vi "Get Shared Variable IP Info.vi"(8 "error in (no error)":errorcluster, 11 "IP Address":string) -> (0 "error out":errorcluster, 3 "Sh Var Data Array":T1[](array[typedef]))   [LabVIEW 2012, in "Shared Variable Custom Device.lvlib"]
uses:
  Shared Variable Custom Device.lvlib
  RTMs/Tree Data.ctl
  <vilib>/Utility/VariantDataType/Type.ctl
  Shared/Shared Variable Globals.vi
  <resource>/objmgr/ni.var.rc
  <vilib>/Utility/VariantDataType/VariantType.lvlib
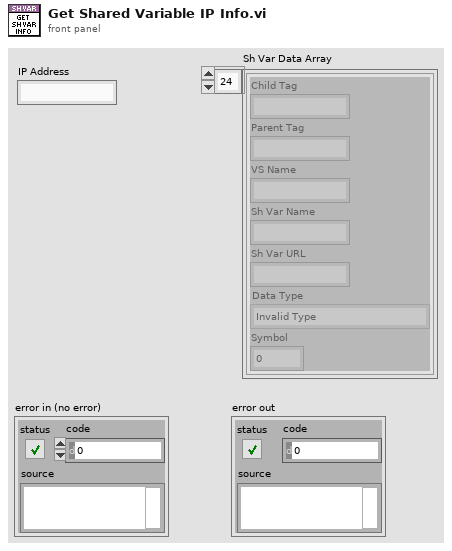
[diagram p1: front panel]
types:
  T1 = typedef "Shared Variable Custom Device.lvlib/Tree Data.ctl" = cluster{"Child Tag":string, "Parent Tag":string, "VS Name":string, "Sh Var Name":string, "Sh Var URL":string, "Data Type":T2, "Symbol":i32}
  T2 = typedef "VariantType.lvlib/Type.ctl" = enum8{"Invalid Type", "Void", "I8", "I16", "I32", "I64", "U8", "U16", "U32", "U64", "Single Float", "Double Float", "Extended Float", "Single Complex", "Double Complex", "Extended Complex", "Enum U8", "Enum U16", "Enum U32", "Enum U64", "Single Float With Unit", "Double Float With Unit", "Extended Float With Unit", "Single Complex with Unit", "Double Complex with Unit", "Extended Complex with Unit", "Boolean", "String", "Path", "Picture", "Tag", "Array", "Cluster", "Variant", "LV Variant", "Waveform", "Timestamp", "Digital Waveform", "Digital Data", "ExpressData", "Refnum", "External Data", "VI", "Poly VI", "LabVIEW Class Instance", "Fixed Point"}
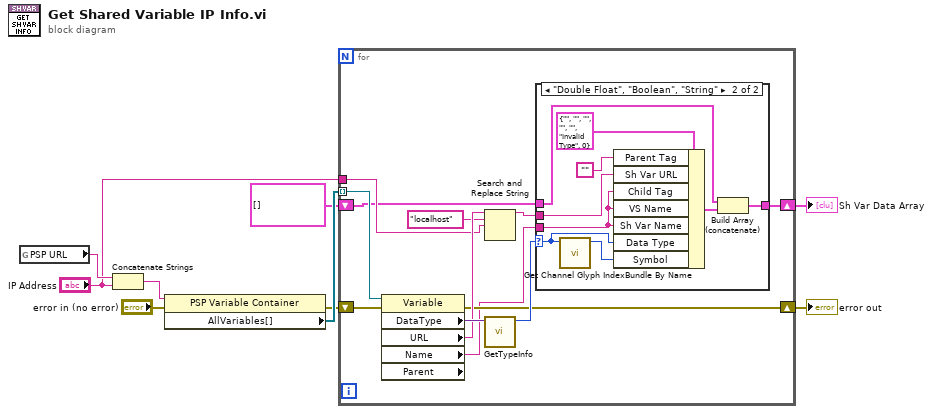
[diagram p0: block diagram]
diagram:
  n1 = global read "Shared Variable Globals.vi" "PSP URL"() -> (w7:string)
  n2 = Concatenate Strings(w7, "IP Address") -> (w3:string)
  n3 = property class="PSP Variable Container"(reference=w3, error in="error in (no error)") -> (error out=w8:errorcluster, "AllVariables[]"=w9:refnum<k21>[])  [unwired: 1 out]
  n4 = for {
    tunnel: w9 -> [w20] mode=indexing
    shift-right: [w14] -> w5
    shift-left: w8 -> [w21]
    tunnel: "IP Address" -> [w16]
    shift-right: [w12] -> w1
    shift-left: T1[] [] ("Sh Var Data Array") -> [w13]
    n5 = property class="Variable" props=["DataType", "URL", "Name", "Parent"](reference=w20, error in=w21) -> (error out=w14:errorcluster, "DataType"=w19:variant, "URL"=w18:string, "Name"=w11:string)  [unwired: 2 out]
    n6 = Search and Replace String(input string=w18, search string="localhost", replace string=w16) -> (result string=w10:string)  [unwired: 5 in, 3 out]
    n7 = call <vilib>:"GetTypeInfo.vi"("Variant"=w19) -> ("Type Enum"=w15:T2)  [unwired: 6 in, 4 out]
    n8 = case shown="\"Double Float\", \"Boolean\", \"String\"" w15 {
      selector: w15 -> [_ w26]
      tunnel: w13 -> [w22 w31]
      tunnel: [w22 w30] -> w12
      tunnel: w11 -> [_ w24]
      tunnel: w10 -> [_ w23]
      frame Default {
      }
      frame "Double Float", "Boolean", "String" {
        n9 = call "Get Channel Glyph Index.vi"("Channel Type"=w26) -> ("Glyph Index"=w27:i32)  [unwired: 10 in]
        n10 = Bundle By Name(cluster=T1 {"Child Tag"="", "Parent Tag"="", "VS Name"="", "Sh Var Name"="", "Sh Var URL"="", "Data Type"=enum."Invalid Type", "Symbol"=0} ("Tree Data"), "Parent Tag"="", "Sh Var URL"=w23, "Child Tag"=w24, "VS Name"=w24, "Sh Var Name"=w24, "Data Type"=w26, "Symbol"=w27) -> (w28:T1)
        n11 = Build Array (concatenate)(w31, w28) -> (w30:T1[])
      }
    }
  }
  "error out" <- w5
  "Sh Var Data Array" <- w1
